vi "Read configuration.vi"(7 "force loading?":bool=TRUE, 8 "error in (no error)":errorcluster, 11 "wavefront sensor in":refnum<class "wavefront sensor.lvclass">) -> (0 "error out":errorcluster, 3 "wavefront sensor out":refnum<class "wavefront sensor.lvclass">)   [LabVIEW 2012, in "wavefront sensor.lvclass"]
doc: "Reads the XML-based configuration file and populates the configuration cluster accordingly. Configuration file name is <component ID>.xml."
uses:
  wavefront sensor.lvclass
  <vilib>/Distrio/Murmex/Murmex/Murmex.lvclass
  wavefront sensor.lvclass/wavefront sensor.ctl
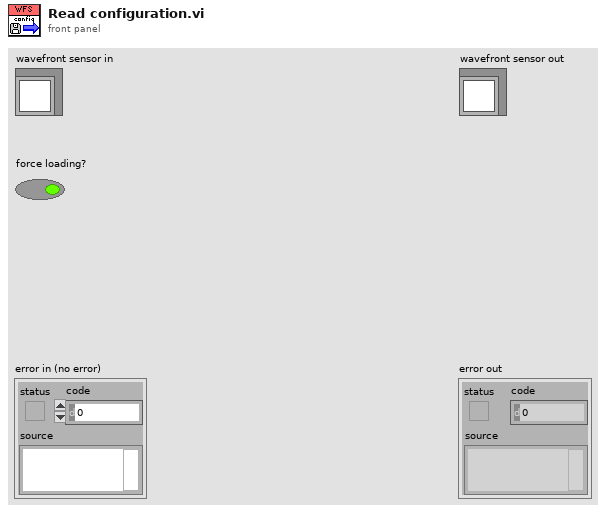
[diagram p1: front panel]
types:
  T1 = typedef "wavefront sensor.lvclass/configuration.ctl" = cluster{"Numeric":dbl}
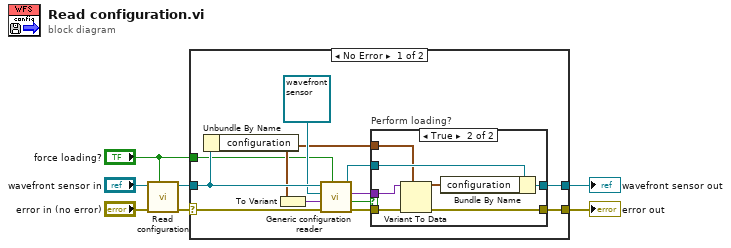
[diagram p0: block diagram]
diagram:
  n1 = call-parent "Read configuration.vi"("force loading?"="force loading?", "error in (no error)"="error in (no error)", "Murmex in"="wavefront sensor in") -> ("error out"=w5:errorcluster, "Murmex out"=w3:refnum<class "wavefront sensor.lvclass">)  [unwired: 7 in]
  n2 = case shown="No Error" w5 {
    selector: w5 -> [w18 w29]
    tunnel: [w16 w29] -> w4
    tunnel: w3 -> [w15 w30]
    tunnel: [w10 w30] -> w2
    tunnel: "force loading?" -> [w8 _]
    frame No Error {
      n3 = Unbundle By Name(w15) -> ("configuration"=w9:T1)
      n4 = To Variant(anything=w9) -> (Variant=w19:variant)
      n5 = call <vilib>:"Generic configuration reader.vi"("force loading?"=w8, "error in (no error)"=w18, "configuration cluster variant"=w19, "inheritance level"=refnum<class "wavefront sensor.lvclass"> refnum ("wavefront sensor"), "Murmex in"=w15) -> ("error out"=w17:errorcluster, "loaded?"=w12:bool, "configuration data (variant)"=w11:variant, "Murmex out"=w13:refnum<class "wavefront sensor.lvclass">)  [unwired: 3 in]
      n6 = case "Perform loading?" shown="True" w12 {
        tunnel: [w21 w24] -> w10
        tunnel: [w20 w28] -> w16
        tunnel: w17 -> [w20 w26]
        tunnel: w13 -> [w21 w27]
        tunnel: w11 -> [_ w25]
        tunnel: w9 -> [_ w23]
        frame False {
        }
        frame True {
          n7 = Variant To Data(error in=w26, type=w23, Variant=w25) -> (data=w22:T1, error out=w28:errorcluster)
          n8 = Bundle By Name(cluster=w27, "configuration"=w22) -> (w24:refnum<class "wavefront sensor.lvclass">)
        }
      }
    }
    frame Error {
    }
  }
  "error out" <- w4
  "wavefront sensor out" <- w2
